vi "Read Weather Forecast Data.vi"(8 "error in (no error)":errorcluster, 11 "Weather in":refnum<class "Weather.lvclass">) -> (0 "error out":errorcluster, 2 "Weather Forecast Data":refnum<vi>, 3 "Weather out":refnum<class "Weather.lvclass">)   [LabVIEW 2025, in "Weather Actor.lvlib" / "Weather.lvclass"]
uses:
  Weather.lvclass
  Weather.lvclass/Weather.ctl
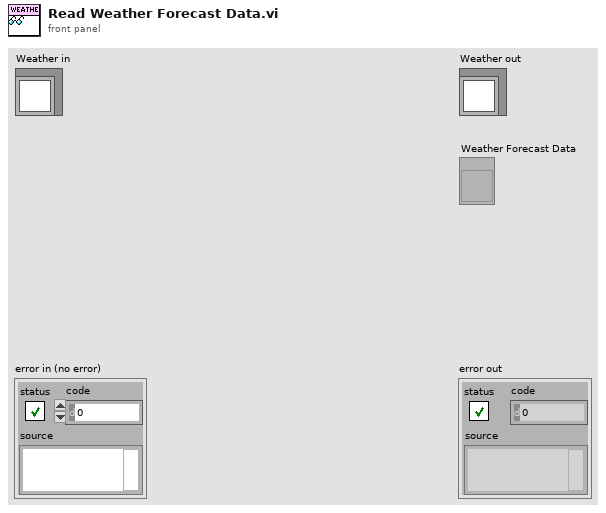
[diagram p1: front panel]
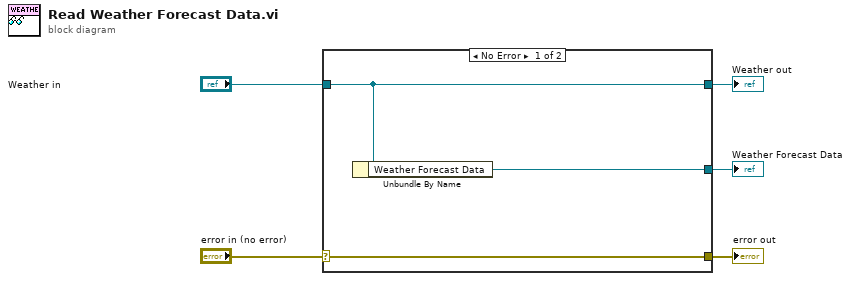
[diagram p0: block diagram]
diagram:
  n1 = case shown="No Error" "error in (no error)" {
    selector: "error in (no error)" -> [w8 w9]
    tunnel: [w8 w9] -> w4
    tunnel: [w7 w10] -> w2
    tunnel: "Weather in" -> [w7 w10]
    tunnel: [w6 _] -> w1
    frame No Error {
      n2 = Unbundle By Name(w7) -> ("Weather Forecast Data"=w6:refnum<vi>)
    }
    frame Error {
    }
  }
  "error out" <- w4
  "Weather out" <- w2
  "Weather Forecast Data" <- w1
